vi "ranged-loop.vi"() -> ()   [LabVIEW 2025]
uses:
  <vilib>/numeric/Random Number (Range) U64.vi
  <vilib>/numeric/sub_Random U32.vi
panel:
  out "indicator":i64
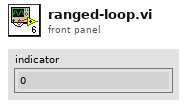
[diagram p1: front panel]
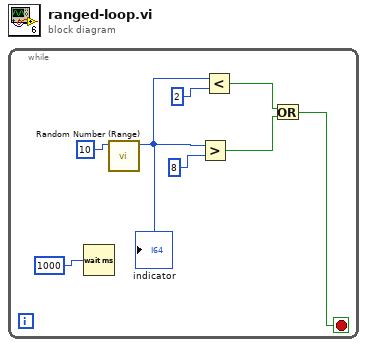
[diagram p0: block diagram]
diagram:
  n1 = while {
    stop <- w2 stop-if-true
    n2 = Wait (ms)(milliseconds to wait=1000) -> ()  [unwired: 1 out]
    n3 = call-poly <vilib>:"Random Number (Range).vi"("upper bound (100)"=10) -> ("number"=w6:u64)  [unwired: 10 in]
    "indicator" <- w6
    n4 = Greater?(x=w6, y=8) -> (0:w3:bool)
    n5 = Less?(x=w6, y=2) -> (x < y?=w4:bool)
    n6 = Or(x=w4, y=w3) -> (x .or. y?=w2:bool)
  }
